vi "AES Angle Processing Unit.vi"(6 "APU.Start Angle":fxp<+,61,10> format="%.55g", 7 "APU.Reset":bool, 11 "APU.Degrees per Tick":fxp<+/-,47,-4>) -> (2 "APU.Cycle Angle":fxp<+,61,10> format="%#.10g", 3 "APU.Crank Angle":fxp<+,60,9> format="%#_10g")   [LabVIEW 2010, in "AES.lvlib" / "AES FPGA.lvlib"]
doc: "Generates two angle values. Cycle angle is from 0-720 degrees. Crank angle is from 0-360 degrees."
uses:
  AES FPGA.lvlib
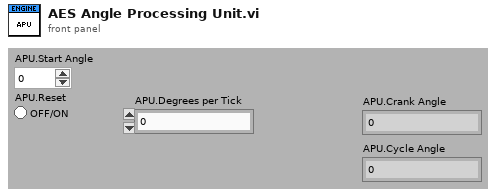
[diagram p1: front panel]
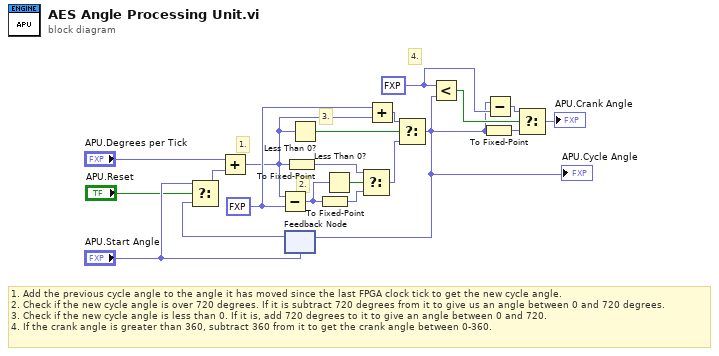
[diagram p0: block diagram]
diagram:
  w11 = fxp<+,6,9> 360.0 ("degrees per crank tick")
  w12 = fxp<+,6,10> 720.0 ("degrees per crank tick")
  # "4."
  # "3."
  # "1. Add the previous cycle angle to the angle it has moved since the last FPGA clock tick to get the new cycle angle.\n2. Check if the new cycle angle is over 720 degrees. If it is subtract 720 degrees from it to give us an angle between 0 and 720 degrees.\n3. Check if the new cycle angle is less than 0. If it is, add 720 degrees to it to give an angle between 0 and 720.\n4. If the crank angle is greater than 360, subtract 360 from it to get the crank angle between 0-360."
  # "2."
  # "1."
  n1 = feedback #1("APU.Start Angle") -> (w4:fxp<+,61,10>)
  n2 = Select(t="APU.Start Angle", s="APU.Reset", f=w4) -> (s? t:f=w3:fxp<+,61,10>)
  n3 = Add(x="APU.Degrees per Tick", y=w3) -> (x+y=w8:fxp<+/-,62,11>)
  n4 = Subtract(x=w8, y=w12) -> (x-y=w6:fxp<+/-,62,11>)
  n5 = To Fixed-Point(number=w8) -> (fixed-point=w10:fxp<+,61,10>)  [unwired: 1 in]
  n6 = Less Than 0?(x=w8) -> (x < 0?=w17:bool)
  n7 = To Fixed-Point(number=w6) -> (fixed-point=w5:fxp<+,61,10>)  [unwired: 1 in]
  n8 = Less Than 0?(x=w6) -> (x < 0?=w19:bool)
  n9 = Select(t=w10, s=w19, f=w5) -> (s? t:f=w9:fxp<+,61,10>)
  n10 = Add(x=w12, y=w8) -> (x+y=w15:fxp<+,61,10>)
  n11 = Select(t=w15, s=w17, f=w9) -> (s? t:f=w7:fxp<+,61,10>)
  "APU.Cycle Angle" <- w7
  n12 = feedback-in #1(w7) -> ()
  n13 = Less?(x=w11, y=w7) -> (x < y?=w16:bool)
  n14 = To Fixed-Point(number=w7) -> (fixed-point=w13:fxp<+,60,9>)  [unwired: 1 in]
  n15 = Subtract(x=w7, y=w11) -> (x-y=w20:fxp<+,60,9>)
  n16 = Select(t=w20, s=w16, f=w13) -> (s? t:f=→"APU.Crank Angle":fxp<+,60,9>)
